vi "Write demandRotatorPositions.vi"(8 "error in (no error)":errorcluster, 10 "RotatorPositions.lvclass":refnum<class "RotatorPositions.lvclass">, 11 "PointingPositions in":refnum<class "PointingPositions.lvclass">) -> (0 "error out":errorcluster, 3 "PointingPositions out":refnum<class "PointingPositions.lvclass">)   [LabVIEW 2014, in "TCSDataDefinitions.lvlib" / "TCSPublicStatus.lvlib" / "PointingPositions.lvlib" / "PointingPositions.lvclass"]
uses:
  PointingPositions.lvclass
  RotatorPositions/RotatorPositions.lvclass
  PointingPositions.lvclass/PointingPositions.ctl
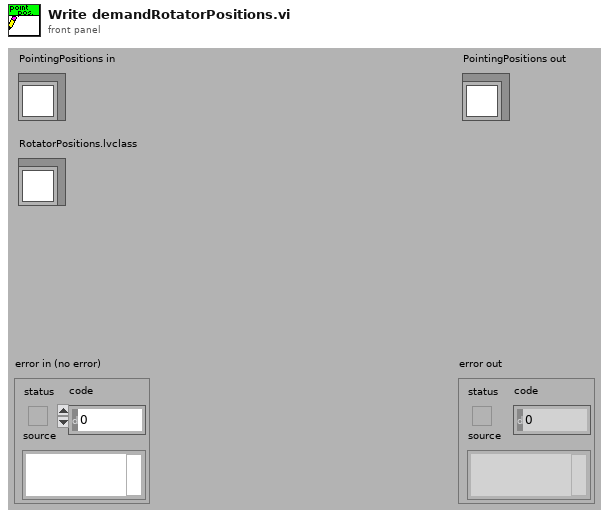
[diagram p1: front panel]
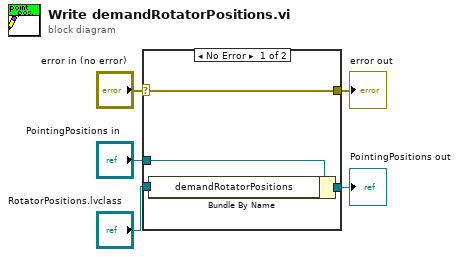
[diagram p0: block diagram]
diagram:
  n1 = case shown="No Error" "error in (no error)" {
    selector: "error in (no error)" -> [w9 w10]
    tunnel: [w9 w10] -> w4
    tunnel: [w7 w11] -> w2
    tunnel: "PointingPositions in" -> [w8 w11]
    tunnel: "RotatorPositions.lvclass" -> [w6 _]
    frame No Error {
      n2 = Bundle By Name(cluster=w8, "demandRotatorPositions"=w6) -> (w7:refnum<class "PointingPositions.lvclass">)
    }
    frame Error {
    }
  }
  "error out" <- w4
  "PointingPositions out" <- w2
